vi "Wait until button is pressed.vi"(6 "Button Info":refnum<vi>, 8 "error in (no error)":errorcluster, 11 "device ID in":refnum<k1>) -> (0 "error out":errorcluster, 3 "Device ID out":refnum<k1>)   [LabVIEW 2014]
uses:
  <vilib>/Utility/inputDevices.llb/joystickAcquire.vi
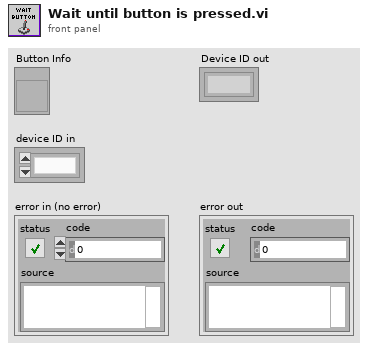
[diagram p1: front panel]
types:
  T1 = cluster{"button 1":bool, "button 2":bool, "button 3":bool, "button 4":bool, "button 5":bool, "button 6":bool, "button 7":bool, "button 8":bool, "button 9":bool, "button 10":bool, "button 11":bool, "button 12":bool, "button 13":bool, "button 14":bool, "button 15":bool, "button 16":bool, "button 17":bool, "button 18":bool, "button 19":bool, "button 20":bool, "button 21":bool, "button 22":bool, "button 23":bool, "button 24":bool, "button 25":bool, "button 26":bool, "button 27":bool, "button 28":bool, "button 29":bool, "button 30":bool, "button 31":bool, "button 32":bool}
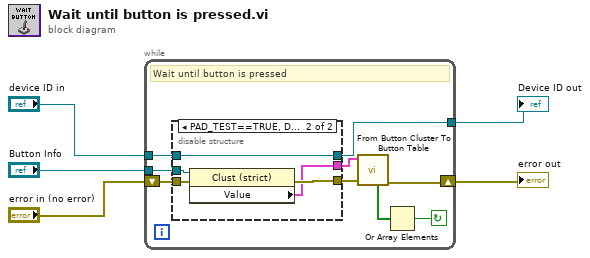
[diagram p0: block diagram]
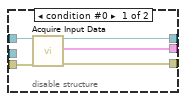
[diagram p2: hidden frame]
diagram:
  n1 = while {
    shift-right: [w12] -> w3
    shift-left: "error in (no error)" -> [w11]
    tunnel: "device ID in" -> [w9]
    tunnel: [w8] -> w5
    tunnel: "Button Info" -> [w7]
    stop <- w13 continue-if-true
    # "Wait until button is pressed"
    n2 = disable-structure shown="PAD_TEST==TRUE, Default" {
      disable-tunnel: w11 -> [w19 w23]
      disable-tunnel: w9 -> [w18 w24]
      disable-tunnel: [w17 w24] -> w8
      disable-tunnel: [w16 w20] -> w6
      disable-tunnel: [w15 w22] -> w10
      disable-tunnel: w7 -> [_ w21]
      frame condition #0 {
        n3 = call-poly <vilib>:"Acquire Input Data.vi"("device ID"=w18, "error in (no error)"=w19) -> ("device ID"=w17:refnum<k1>, "button info"=w16:T1, "error out"=w15:errorcluster)  [unwired: 13 in, 2 out]
      }
      frame condition #1 (active) {
        n4 = property on="Property Node" class="Clust (strict)"(reference=w21, error in=w23) -> (error out=w22:errorcluster, "Value"=w20:T1)  [unwired: 1 out]
      }
    }
    n5 = call "From Button Cluster To Button Table.vi"("Error In"=w10, "button info"=w6) -> ("Error Out"=w12:errorcluster, "Buttons array"=w14:bool[])  [unwired: 7 in, 1 out]
    n6 = Or Array Elements(Boolean array=w14) -> (logical OR=w13:bool)
  }
  "Device ID out" <- w5
  "error out" <- w3
